vi "Get gRPC Package.vi"(8 "error in (no error)":errorcluster, 11 "protoFile ref in":u64) -> (0 "error out":errorcluster, 2 "Package ref  out":u64, 3 "protoFile ref out":u64)   [LabVIEW 2019, in "gRPC Scripting Tools.lvlib"]
uses:
  gRPC Scripting Tools.lvlib
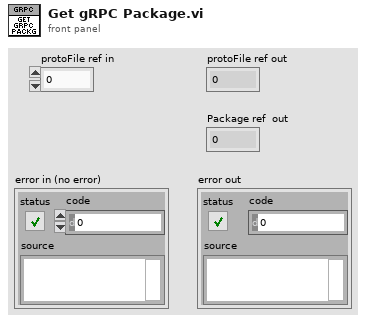
[diagram p1: front panel]
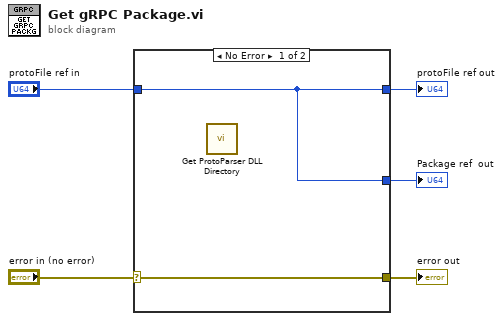
[diagram p0: block diagram]
diagram:
  n1 = case shown="No Error" "error in (no error)" {
    selector: "error in (no error)" -> [w7 w9]
    tunnel: "protoFile ref in" -> [w6 w8]
    tunnel: [w7 w9] -> w3
    tunnel: [w6 w8] -> w2
    tunnel: [w6 _] -> w1
    frame No Error {
      n2 = call "Get ProtoParser DLL Directory.vi"() -> ()  [unwired: 1 out]
    }
    frame Error {
    }
  }
  "error out" <- w3
  "protoFile ref out" <- w2
  "Package ref  out" <- w1
